vi "Do.vi"(8 "error in (no error)":errorcluster, 10 "Actor in":refnum<class "Actor.lvclass">, 11 "Update Cache Msg in":refnum<class "Update Cache Msg.lvclass">) -> (0 "error out":errorcluster, 2 "Actor out":refnum<class "Actor.lvclass">)   [LabVIEW 2023, in "Class Loader.lvlib" / "Update Cache Msg.lvclass"]
doc: "(<B>Filename</B>: Actor Framework.lvlib:Message.lvclass:Do.vi)\n\nDefines what a message does when it is received by an actor. Generally, a message instructs an actor to invoke one of its methods. By default, this method does nothing. A child class must override it to define behavior. Create a child class by using the Actor Framework Message Maker dialog box."
uses:
  Update Cache Msg.lvclass
  <vilib>/ActorFramework/Actor/Actor.lvclass
  Class Loader/Class Loader.lvclass
  C:/Program Files/National Instruments/LabVIEW 2025/vi.lib/ActorFramework/Actor/Actor.lvclass
  Update Cache Msg.lvclass/Update Cache Msg.ctl
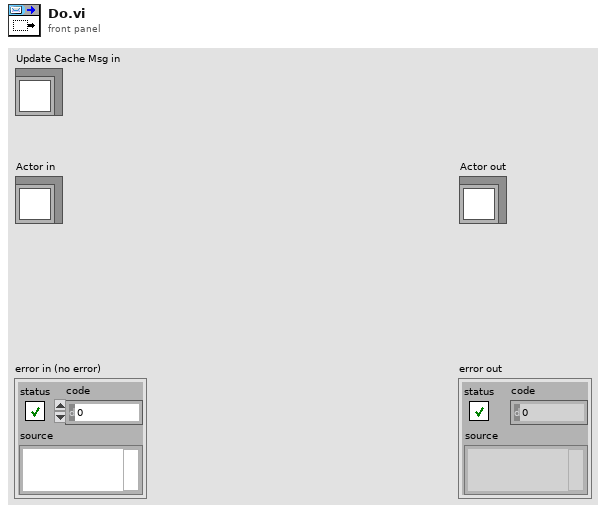
[diagram p1: front panel]
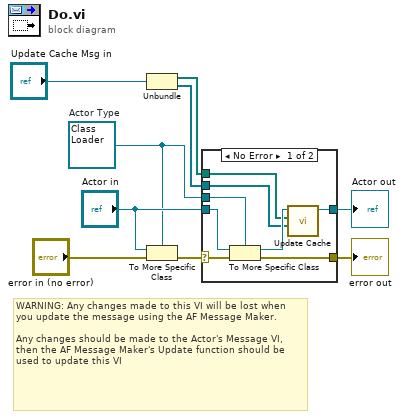
[diagram p0: block diagram]
diagram:
  w4 = refnum<class "Class Loader.lvclass"> refnum  # Actor Type
  # "WARNING: Any changes made to this VI will be lost when you update the message using the AF Message Maker.\n\nAny changes should be made to the Actor's Message VI, then the AF Message Maker's Update function should be used to update this VI"
  n1 = Unbundle("Update Cache Msg in") -> (w3:path[], w2:refnum<class>[])
  n2 = To More Specific Class(target class=w4, reference="Actor in", error in="error in (no error)") -> (error out=w8:errorcluster)  [unwired: 1 out]
  n3 = case shown="No Error" w8 {
    selector: w8 -> [w17 w19]
    tunnel: [w13 w19] -> w7
    tunnel: [w12 w18] -> w6
    tunnel: "Actor in" -> [w16 w18]
    tunnel: w4 -> [w15 _]
    tunnel: w3 -> [w11 _]
    tunnel: w2 -> [w10 _]
    frame No Error {
      n4 = To More Specific Class ("Actor Cast")(target class=w15, reference=w16, error in=w17) -> (specific class reference=w14:refnum<class "Class Loader.lvclass">, error out=w13:errorcluster)
      n5 = call "Update Cache.vi"("Classes"=w10, "Paths"=w11, "Class Loader in"=w14) -> ("Class Loader out"=w12:refnum<class "Class Loader.lvclass">)  [unwired: 8 in]
    }
    frame Error {
    }
  }
  "error out" <- w7
  "Actor out" <- w6
